vi "Move servo to angle (SG90 180 degrees).vi"(8 "Position":dbl format="%.6f", 10 "Output Terminal":tag="/Dev1/PFI3", 11 "Counter":tag="Dev1/ctr0") -> (0 "Actual Duty Cycle":dbl, 1 "Actual Frequency":dbl)   [LabVIEW 2017]
uses:
  <vilib>/Utility/error.llb/DialogType.ctl
  <vilib>/DAQmx/create/channels.llb/DAQmx Create Channel (CO-Pulse Generation-Frequency).vi
  <vilib>/DAQmx/configure/timing.llb/DAQmx Timing (Implicit).vi
  <resource>/objmgr/daqmx.rc
panel:
  out "Out of Range":bool
  in  "Stop":bool
  # "Channel Settings"
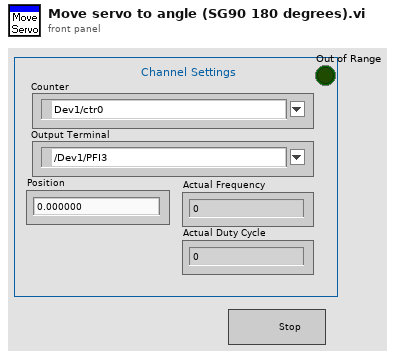
[diagram p1: front panel]
types:
  T1 = typedef "DialogType.ctl" = u16
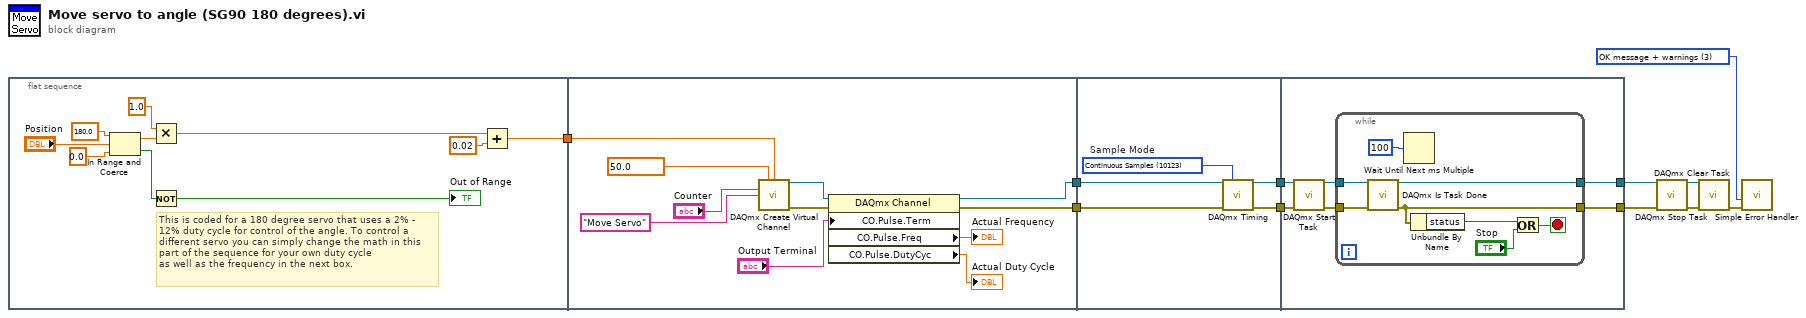
[diagram p0: block diagram]
diagram:
  w2 = T1 3 items=["no dialog", "OK message", "continue or stop message", "OK message + warnings", "continue/stop + warnings"] ("type of dialog (OK msg:1)")
  n1 = flat-sequence {
    tunnel: [w12] -> w1
    tunnel: [w26] -> w11
    tunnel: [w25] -> w10
    tunnel: w1 -> [w22]
    tunnel: w11 -> [w36]
    tunnel: w10 -> [w35]
    tunnel: [w34] -> w9
    tunnel: [w33] -> w8
    tunnel: w9 -> [w41]
    tunnel: w8 -> [w40]
    tunnel: [w39] -> w4
    tunnel: [w38] -> w3
    frame #0 {
      # "This is coded for a 180 degree servo that uses a 2% - 12% duty cycle for control of the angle. To control a different servo you can simply change the math in this part of the sequence for your own duty cycle\nas well as the frequency in the next box."
      n2 = In Range and Coerce(upper limit=180.0, x="Position", lower limit=0.0) -> (coerced(x)=w16:dbl, In Range?=w18:bool)
      n3 = Multiply(x=1.0, y=w16) -> (x*y=w14:dbl)
      n4 = Not(x=w18) -> (.not. x?=→"Out of Range":bool)
      n5 = Add(x=w14, y=0.02) -> (x+y=w12:dbl)
    }
    frame #1 {
      n6 = call-poly <vilib>:"DAQmx Create Virtual Channel.vi"("frequency"=50.0 ("Frequency"), "duty cycle"=w22, "counter"="Counter", "name to assign"="Move Servo") -> ("task out"=w31:refnum<k21>, "error out"=w30:errorcluster)  [unwired: 10 in]
      n7 = property class="DAQmx Channel"(reference=w31, error in=w30, "CO.Pulse.Term"="Output Terminal") -> (reference out=w25:refnum<k21>, error out=w26:errorcluster, "CO.Pulse.Freq"=→"Actual Frequency":dbl, "CO.Pulse.DutyCyc"=→"Actual Duty Cycle":dbl)
    }
    frame #2 {
      w37 = 10123 items=["Finite Samples"=10178, "Continuous Samples"=10123, "Hardware Timed Single Point"=12522]  # Sample Mode
      n8 = call-poly <vilib>:"DAQmx Timing.vi"("task/channels in"=w35, "sample mode"=w37, "error in"=w36) -> ("task out"=w34:refnum<k21>, "error out"=w33:errorcluster)  [unwired: 11 in]
    }
    frame #3 {
      n9 = call <vilib>:"DAQmx Start Task.vi"("task/channels in"=w41, "error in"=w40) -> ("task out"=w42:refnum<k21>, "error out"=w43:errorcluster)  [unwired: 12 in]
      n10 = while {
        tunnel: w42 -> [w51]
        tunnel: w43 -> [w50]
        tunnel: [w45] -> w39
        tunnel: [w44] -> w38
        stop <- w49 stop-if-true
        n11 = call <vilib>:"DAQmx Is Task Done.vi"("task/channels in"=w51, "error in"=w50) -> ("task out"=w45:refnum<k21>, "error out"=w44:errorcluster)  [unwired: 11 in, 1 out]
        n12 = Wait Until Next ms Multiple(millisecond multiple=u32 100) -> ()  [unwired: 1 out]
        n13 = Unbundle By Name(w44) -> ("status"=w48:bool)
        n14 = Or(x=w48, y="Stop") -> (x .or. y?=w49:bool)
      }
    }
  }
  n15 = call <vilib>:"DAQmx Stop Task.vi"("task/channels in"=w4, "error in"=w3) -> ("task out"=w6:refnum<k21>, "error out"=w5:errorcluster)  [unwired: 12 in]
  n16 = call <vilib>:"DAQmx Clear Task.vi"("task in"=w6, "error in"=w5) -> ("error out"=w7:errorcluster)  [unwired: 13 in]
  n17 = call <vilib>:"Simple Error Handler.vi"("type of dialog (OK msg:1)"=w2, "error in (no error)"=w7) -> ()  [unwired: 3 in, 5 out]
